vi "ConvertUnit.vi"(8 "error in":errorcluster, 9 "Desired Unit":string, 10 "Channel Properties":variant, 11 "Value":sgl) -> (0 "error out":errorcluster, 3 "Scaled Value":sgl)   [LabVIEW 2017]
uses:
  <vilib>/addons/_NISVFA/_Shared subVIs/Controls/svc_Engineering Units Text Ring.ctl
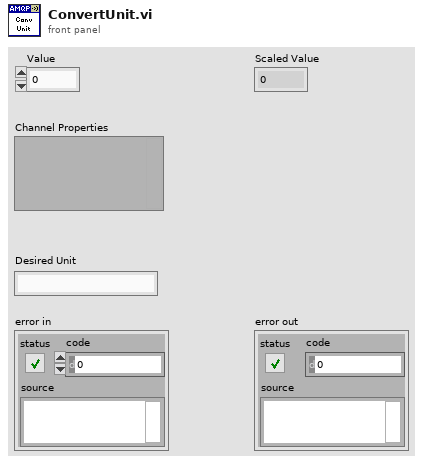
[diagram p1: front panel]
types:
  T1 = typedef "svc_Engineering Units Text Ring.ctl" = u16
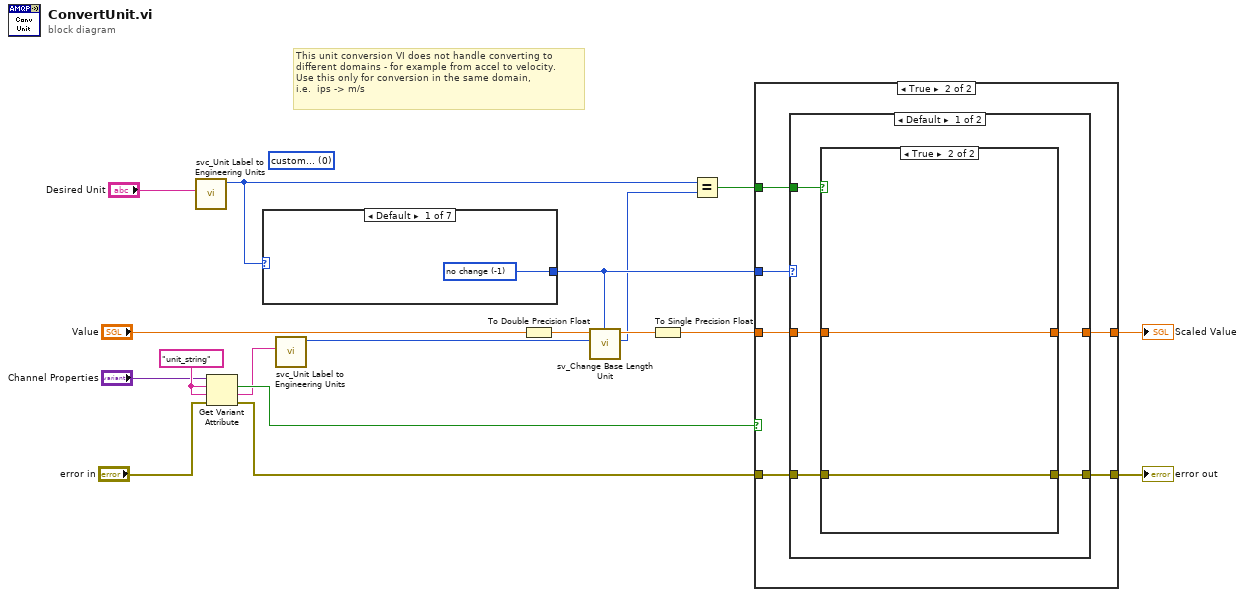
[diagram p0: block diagram]
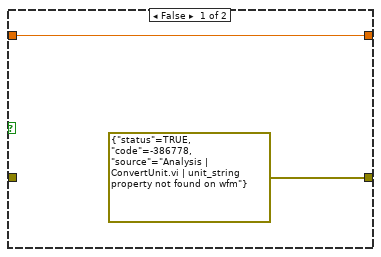
[diagram p2: hidden frame]
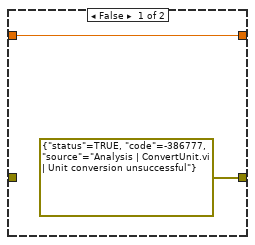
[diagram p3: hidden frame]
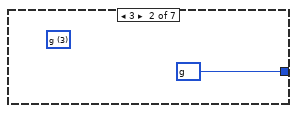
[diagram p5: hidden frame]
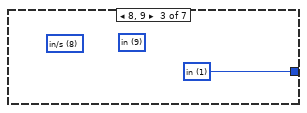
[diagram p6: hidden frame]
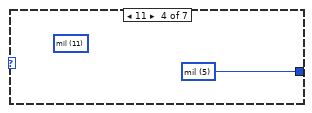
[diagram p7: hidden frame]
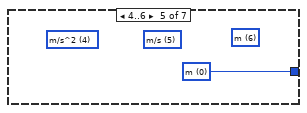
[diagram p8: hidden frame]
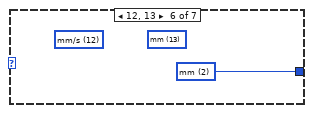
[diagram p9: hidden frame]
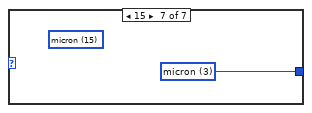
[diagram p10: hidden frame]
diagram:
  (unwired) T1 0 items=["custom..."=0, "V"=1, "A"=21, "Pa"=2, "N"=20, "g"=3, "m/s^2"=4, "m/s"=5, "m"=6, "mm/s"=12, "mm"=13, "micron/s"=14, "micron"=15, "in/s^2"=7, "in/s"=8, "in"=9, "mil/s"=10, "mil"=11, "rad/s^2"=16, "rad/s"=17, "rad"=18, "deg/s^2"=26, "deg/s"=27, "deg"=28, "RPM"=22, "cycle/s^2"=23, "Hz"=24, "cycle"=25, "strain"=19] ("engineering units")
  w18 = "unit_string" ("property name")
  # "This unit conversion VI does not handle converting to\ndifferent domains - for example from accel to velocity.\nUse this only for conversion in the same domain,\ni.e.  ips -> m/s"
  n1 = call <vilib>:"svc_Unit Label to Engineering Units.vi"("unit label"="Desired Unit") -> ("engineering units"=w11:T1)  [unwired: 9 in, 1 out]
  n2 = Get Variant Attribute(Variant="Channel Properties", name=w18, default value (empty Variant)=w18, error in="error in") -> (found=w5:bool, value=w4:string, error out=w2:errorcluster)  [unwired: 1 out]
  n3 = case shown="Default" w11 {
    tunnel: [w19 w20 w21 w22 w23 w24 w25] -> w7
    frame Default {
      w19 = -1 items=["no change"=-1, "g"=386, "m"=0, "cm"=4, "mm"=2, "micron"=3, "in"=1, "mil"=5] ("desired base units for vibration")
    }
    frame 3 {
      w20 = 386 items=["no change"=-1, "g"=386, "m"=0, "cm"=4, "mm"=2, "micron"=3, "in"=1, "mil"=5] ("desired base units for vibration")
      (unwired) T1 3 items=["custom..."=0, "V"=1, "A"=21, "Pa"=2, "N"=20, "g"=3, "m/s^2"=4, "m/s"=5, "m"=6, "mm/s"=12, "mm"=13, "micron/s"=14, "micron"=15, "in/s^2"=7, "in/s"=8, "in"=9, "mil/s"=10, "mil"=11, "rad/s^2"=16, "rad/s"=17, "rad"=18, "deg/s^2"=26, "deg/s"=27, "deg"=28, "RPM"=22, "cycle/s^2"=23, "Hz"=24, "cycle"=25, "strain"=19] ("engineering units")
    }
    frame 8, 9 {
      (unwired) T1 9 items=["custom..."=0, "V"=1, "A"=21, "Pa"=2, "N"=20, "g"=3, "m/s^2"=4, "m/s"=5, "m"=6, "mm/s"=12, "mm"=13, "micron/s"=14, "micron"=15, "in/s^2"=7, "in/s"=8, "in"=9, "mil/s"=10, "mil"=11, "rad/s^2"=16, "rad/s"=17, "rad"=18, "deg/s^2"=26, "deg/s"=27, "deg"=28, "RPM"=22, "cycle/s^2"=23, "Hz"=24, "cycle"=25, "strain"=19] ("engineering units")
      w21 = 1 items=["no change"=-1, "g"=386, "m"=0, "cm"=4, "mm"=2, "micron"=3, "in"=1, "mil"=5] ("desired base units for vibration")
      (unwired) T1 8 items=["custom..."=0, "V"=1, "A"=21, "Pa"=2, "N"=20, "g"=3, "m/s^2"=4, "m/s"=5, "m"=6, "mm/s"=12, "mm"=13, "micron/s"=14, "micron"=15, "in/s^2"=7, "in/s"=8, "in"=9, "mil/s"=10, "mil"=11, "rad/s^2"=16, "rad/s"=17, "rad"=18, "deg/s^2"=26, "deg/s"=27, "deg"=28, "RPM"=22, "cycle/s^2"=23, "Hz"=24, "cycle"=25, "strain"=19] ("engineering units")
    }
    frame 11 {
      w22 = 5 items=["no change"=-1, "g"=386, "m"=0, "cm"=4, "mm"=2, "micron"=3, "in"=1, "mil"=5] ("desired base units for vibration")
      (unwired) T1 11 items=["custom..."=0, "V"=1, "A"=21, "Pa"=2, "N"=20, "g"=3, "m/s^2"=4, "m/s"=5, "m"=6, "mm/s"=12, "mm"=13, "micron/s"=14, "micron"=15, "in/s^2"=7, "in/s"=8, "in"=9, "mil/s"=10, "mil"=11, "rad/s^2"=16, "rad/s"=17, "rad"=18, "deg/s^2"=26, "deg/s"=27, "deg"=28, "RPM"=22, "cycle/s^2"=23, "Hz"=24, "cycle"=25, "strain"=19] ("engineering units")
    }
    frame 4..6 {
      (unwired) T1 6 items=["custom..."=0, "V"=1, "A"=21, "Pa"=2, "N"=20, "g"=3, "m/s^2"=4, "m/s"=5, "m"=6, "mm/s"=12, "mm"=13, "micron/s"=14, "micron"=15, "in/s^2"=7, "in/s"=8, "in"=9, "mil/s"=10, "mil"=11, "rad/s^2"=16, "rad/s"=17, "rad"=18, "deg/s^2"=26, "deg/s"=27, "deg"=28, "RPM"=22, "cycle/s^2"=23, "Hz"=24, "cycle"=25, "strain"=19] ("engineering units")
      (unwired) T1 5 items=["custom..."=0, "V"=1, "A"=21, "Pa"=2, "N"=20, "g"=3, "m/s^2"=4, "m/s"=5, "m"=6, "mm/s"=12, "mm"=13, "micron/s"=14, "micron"=15, "in/s^2"=7, "in/s"=8, "in"=9, "mil/s"=10, "mil"=11, "rad/s^2"=16, "rad/s"=17, "rad"=18, "deg/s^2"=26, "deg/s"=27, "deg"=28, "RPM"=22, "cycle/s^2"=23, "Hz"=24, "cycle"=25, "strain"=19] ("engineering units")
      w23 = 0 items=["no change"=-1, "g"=386, "m"=0, "cm"=4, "mm"=2, "micron"=3, "in"=1, "mil"=5] ("desired base units for vibration")
      (unwired) T1 4 items=["custom..."=0, "V"=1, "A"=21, "Pa"=2, "N"=20, "g"=3, "m/s^2"=4, "m/s"=5, "m"=6, "mm/s"=12, "mm"=13, "micron/s"=14, "micron"=15, "in/s^2"=7, "in/s"=8, "in"=9, "mil/s"=10, "mil"=11, "rad/s^2"=16, "rad/s"=17, "rad"=18, "deg/s^2"=26, "deg/s"=27, "deg"=28, "RPM"=22, "cycle/s^2"=23, "Hz"=24, "cycle"=25, "strain"=19] ("engineering units")
    }
    frame 12, 13 {
      (unwired) T1 13 items=["custom..."=0, "V"=1, "A"=21, "Pa"=2, "N"=20, "g"=3, "m/s^2"=4, "m/s"=5, "m"=6, "mm/s"=12, "mm"=13, "micron/s"=14, "micron"=15, "in/s^2"=7, "in/s"=8, "in"=9, "mil/s"=10, "mil"=11, "rad/s^2"=16, "rad/s"=17, "rad"=18, "deg/s^2"=26, "deg/s"=27, "deg"=28, "RPM"=22, "cycle/s^2"=23, "Hz"=24, "cycle"=25, "strain"=19] ("engineering units")
      w24 = 2 items=["no change"=-1, "g"=386, "m"=0, "cm"=4, "mm"=2, "micron"=3, "in"=1, "mil"=5] ("desired base units for vibration")
      (unwired) T1 12 items=["custom..."=0, "V"=1, "A"=21, "Pa"=2, "N"=20, "g"=3, "m/s^2"=4, "m/s"=5, "m"=6, "mm/s"=12, "mm"=13, "micron/s"=14, "micron"=15, "in/s^2"=7, "in/s"=8, "in"=9, "mil/s"=10, "mil"=11, "rad/s^2"=16, "rad/s"=17, "rad"=18, "deg/s^2"=26, "deg/s"=27, "deg"=28, "RPM"=22, "cycle/s^2"=23, "Hz"=24, "cycle"=25, "strain"=19] ("engineering units")
    }
    frame 15 {
      w25 = 3 items=["no change"=-1, "g"=386, "m"=0, "cm"=4, "mm"=2, "micron"=3, "in"=1, "mil"=5] ("desired base units for vibration")
      (unwired) T1 15 items=["custom..."=0, "V"=1, "A"=21, "Pa"=2, "N"=20, "g"=3, "m/s^2"=4, "m/s"=5, "m"=6, "mm/s"=12, "mm"=13, "micron/s"=14, "micron"=15, "in/s^2"=7, "in/s"=8, "in"=9, "mil/s"=10, "mil"=11, "rad/s^2"=16, "rad/s"=17, "rad"=18, "deg/s^2"=26, "deg/s"=27, "deg"=28, "RPM"=22, "cycle/s^2"=23, "Hz"=24, "cycle"=25, "strain"=19] ("engineering units")
    }
  }
  n4 = call <vilib>:"svc_Unit Label to Engineering Units.vi"("unit label"=w4) -> ("engineering units"=w15:T1)  [unwired: 9 in, 1 out]
  n5 = To Double Precision Float(number="Value") -> (double precision float=w13:dbl)
  n6 = call <vilib>:"sv_Change Base Length Unit.vi"("desired base units for vibration"=w7, "engineering units in"=w15, "value in [EU]"=w13) -> ("engineering units out"=w1:T1, "value out [desired EU]"=w12:dbl)  [unwired: 4 in, 1 out]
  n7 = To Single Precision Float(number=w12) -> (single precision float=w9:sgl)
  n8 = Equal?(x=w11, y=w1) -> (x = y?=w6:bool)
  n9 = case shown="True" w5 {
    tunnel: [w27 w31] -> w10
    tunnel: w9 -> [w27 w30]
    tunnel: [errorcluster {"status"=TRUE, "code"=-386778, "source"="Analysis | ConvertUnit.vi | unit_string property not found on wfm"} ("error out") w32] -> w8
    tunnel: w7 -> [_ w33]
    tunnel: w6 -> [_ w29]
    tunnel: w2 -> [_ w28]
    frame False {
    }
    frame True {
      n10 = case shown="Default" w33 {
        tunnel: [w35 w43] -> w32
        tunnel: [w37 w44] -> w31
        tunnel: w30 -> [w36 w44]
        tunnel: w29 -> [w38 _]
        tunnel: w28 -> [w34 w43]
        frame Default {
          n11 = case shown="True" w38 {
            tunnel: [w40 w42] -> w37
            tunnel: w36 -> [w40 w42]
            tunnel: [errorcluster {"status"=TRUE, "code"=-386777, "source"="Analysis | ConvertUnit.vi | Unit conversion unsuccessful"} ("error out") w41] -> w35
            tunnel: w34 -> [_ w41]
            frame False {
            }
            frame True {
            }
          }
        }
        frame -1 {
          # "no change in units"
        }
      }
    }
  }
  "Scaled Value" <- w10
  "error out" <- w8
